vi "Get Max Nested Level To Go.vi"() -> (0 "max nested level":i32=42)   [LabVIEW 2014]
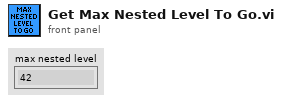
[diagram p1: front panel]
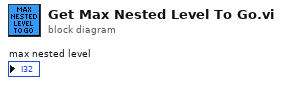
[diagram p0: block diagram]
diagram:
